vi "STOP.vi"(8 "error in (no error)":errorcluster, 11 "Stop in":refnum<class "STREAK_camera.lvclass">) -> (0 "error out":errorcluster, 3 "Stop out":refnum<class "STREAK_camera.lvclass">)   [LabVIEW 2019, in "STREAK_camera.lvclass"]
uses:
  STREAK_camera.lvclass
  Detector.lvclass
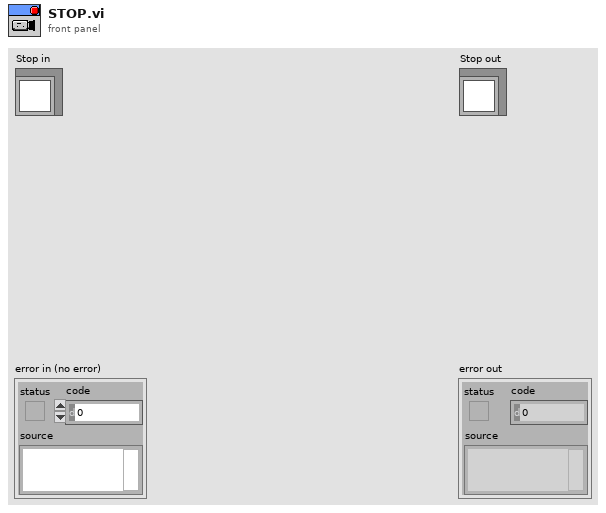
[diagram p1: front panel]
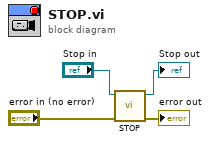
[diagram p0: block diagram]
diagram:
  n1 = call-parent "STOP.vi"("error in (no error)"="error in (no error)", "Stop in"="Stop in") -> ("error out"=→"error out":errorcluster, "Stop out"=→"Stop out":refnum<class "STREAK_camera.lvclass">)  [unwired: 8 in]
